vi "HFRR ADV v01.vi"() -> ()   [LabVIEW 2025] (continued)
  # "mm"
  # "°C"
  # "%RH"
  # "min"
  # "mins remaining"
  # "°C"
  # "Coefficient of Friction"
  # "Frictional Force ( N )"
  # "Electrical Contact Resistance ( % )"
  # "Temperature ( °C )"
  # "Heater"
  # "( mm )"
  # "Hz"
  # "%Rh"
  # "Stroke ( mm )"
  # "Controller"
  # "%"
  # "N"
  # "deg C"
  # "N"
  # "Automated Scar Detection in Progress"
  # "Zoom Factor"
  # "%"
  # "Tools"
  # "Wear Scar Measurements"
  # "Wear Scar"
  # "Wear Scar"
  # "Wear Scar"
  # "µm"
  # "µm"
  # "µm"
  # "Calibration Centre\nSelect a calibration procedure to begin. Each procedure guides you through all required steps."
  # "LAST CALIBRATION SESSION"
  # "Stroke"
  # "Friction"
  # "Temperature"
  # "Apply known deadweight loads to validate \nthe friction force measurement chain \nand compute the calibration factor for the f\norce transducer."
  # "Step-by-step guided displacement calibration \nacross 6 positions from 0.1 mm to 1.2 mm. Tear \nfirst, then measure each position one by one."
  # "Two-set calibration: one point at 0 °C \nice-point) and one at 60 °C (high-point) \nusing a  reference Calibrator."
  # "Step 1 — Ball Holder"
  # "Remove the ball holder by loosening and removing the center screw for stroke calibration."
  # "Step 2 — Disc Holder"
  # "Remove the disc holder by loosening and removing the screws. Clean any fluid present in the disc holder."
  # "Step 3 — Calibration Head"
  # "Place the calibration holder in position and securely tighten the center screw."
  # "Step 4 — Calibration Holder"
  # "Place the calibration holder in position and tighten the two securing screws"
  # "Step 5 — Calibration Carriage"
  # "Position the calibration carriage in the center cavity of the calibration holder and securely tighten the upper and side screws"
  # "Step 7 — Tare ( ZERO REFERENCE )"
  # "Move the carriage to the mechanical zero stop — no displacement applied. Before measuring, the sensor must be Preset. Once in position, tap Tare & Begin to zero the reference."
  # "Step 8 — POSITION MEASUREMENT"
  # "Measurement Checklist"
  # "Position the carriage at exactly this \nvalue using your reference gauge, then tap Confirm &\n Next."
  # "Positions recorded!\n\nTap Confirm & Next  to review the calibration summary."
  # "Step 9 — CALIBRATION RESULT"
  # "Stroke Calibration Complete"
  # "Calibration completed successfully. The measured stroke length is within the acceptable tolerance range of the factory calibration value."
  # "Calibration failed. The measured stroke length differs from the factory calibration value by more than 20%. Please perform the calibration again."
  # "Step 1 — Ball Holder"
  # "Remove the ball holder by loosening and removing the center screw for Friction calibration."
  # "Step 2 — Disc Holder"
  # "Remove the disc holder by loosening and removing the opposing screws. Clean any fluid present in the disc holder."
  # "Step 3 — Calibration Head"
  # "Place the calibration holder in position and securely tighten the center screw."
  # "Step 4 — Calibration Holder"
  # "Place the calibration holder in position and tighten the two securing screws"
  # "Step 5 — Tare (Spring at Free Length)"
  # "Ensure the spring is at its contact (compressed) length — the micrometer head is in contact. Click Tare Sensor to zero the friction force baseline."
  # "Step 6 — Measure Friction Force"
  # "Run the Actual Test to measure Friction Force."
  # "Calibration in Progress"
  # "Step 7 — CALIBRATION RESULT"
  # "Calibration completed successfully. The measured friction force is within the acceptable tolerance range of the factory calibration value."
  # "Calibration failed. The measured friction force differs from the factory calibration value . Please perform the calibration again."
  # "Spring Constant: k = 1.000 N/mm\nSpring force |F| = k Ч d"
  # "Calibrates the sample/bath temperature sensor. \nUsed for test specimen and lubricant temperature measurement."
  # "Calibrates the ambient air temperature sensor. \nUsed for environmental chamber monitoring."
  # "Set B\n60 °C\nHigh-point calibration"
  # "Set A\n0 °C\nIce-point calibration"
  # "Set B\n60 °C\nHigh-point calibration"
  # "Set A\n0 °C\nIce-point calibration"
  # "Select Temperature Sensor"
  # "Choose which temperature sensor you are calibrating. Both use the same two-\npoint procedure: 0 °C (ice-point) and 60 °C (high-point)."
  # "Step 1 — Reference Instrument Setup"
  # "Connect a calibrated reference to the DUT port. This calibration performs two sets: one at 0 °C and one at 60 °C."
  # "Set A\n0 °C\nIce-point calibration"
  # "Set B\n60 °C\nHigh-point calibration"
  # "Allow the temperature bath to stabilise for at least 2 minutes at each set-point before recording the reading."
  # "Step 2 — Set A:  0 °C Calibration"
  # "Connect the  0 °C reference connector. Wait for the temperature to stabilise. Once stable, and click Record Point."
  # "Step 3 — Set B:  60 °C Calibration"
  # "Connect the  60 °C reference connector. Wait for the temperature to stabilise. Once stable, and click Record Point."
  # "Sample Temperature Calibration Complete"
  # "Sample Temperature Calibration PASSED\nMax deviation 0.200 °C — within ±0.5 °C tolerance. Two-point correction applied (0 °C & 60 °C)."
  # "Sample  Temperature Calibration Failed\nmeasured Sample Temperature differs from the factory calibration value"
  # "Step 1 — Reference Instrument Setup"
  # "Connect a calibrated reference to the DUT port. This calibration performs two sets: one at 0 °C and one at 60 °C."
  # "Set A\n0 °C\nIce-point calibration"
  # "Set B\n60 °C\nHigh-point calibration"
  # "Allow the temperature bath to stabilise for at least 2 minutes at each set-point before recording the reading."
  # "Step 2 — Set A:  0 °C Calibration"
  # "Connect the  0 °C reference connector. Wait for the temperature to stabilise. Once stable, and click Record Point."
  # "Step 3 — Set B:  60 °C Calibration"
  # "Connect the  60 °C reference connector. Wait for the temperature to stabilise. Once stable, and click Record Point."
  # "Air Temperature Calibration Complete"
  # "Air Temperature Calibration PASSED\nMax deviation 0.200 °C — within ±0.5 °C tolerance. Two-point correction applied (0 °C & 60 °C)."
  # "Air  Temperature Calibration Failed\nmeasured Sample Temperature differs from the factory calibration value"
  # "PID SAVE PARAMETERS"
  # "STROKE CALIBRATION"
  # "FF CALIBRATION"
  # "ABOUT SCREEN SAVE PARAMETERS"
  # "© 2023"
  # "System Control Commands\nS;1 - Starts the full automation cycle (Runs Priming-humidify till 70RH sequence first, then switches to Maintenance).\nS;0 - Stops the system immediately and enters Standby mode (Safe State: All actuators OFF).\nM;1 - Skips the priming sequence and jumps directly to Maintenance mode (PID control).\nR;1 - Resets the logic state machine and clears all errors, returning to Standby.\nService Mode (Manual Control)\nX;1 - Enters Manual Service Mode. This disables all automatic logic, sensor safety checks, and timers.\nX;0 - Exits Manual Service Mode and returns to Standby (Safe State).\nActuator Commands (Only work after sending X;1)\nP;[0-255] - Sets the Pump PWM. Note that this is Active Low (0 = Max Flow, 255 = Pump OFF).\nF;I;[0-255] - Sets the Intake Fan speed (0 = OFF, 255 = Max Speed).\nF;O;[0-255] - Sets the Exhaust Fan speed (0 = OFF, 255 = Max Speed).\nD;1 - Turns the Dehumidifier Relay ON.\nD;0 - Turns the Dehumidifier Relay OFF."
  # "%RH"
types:
  T1 = enum32{"Home", "Dashboard", "Imaging", "Report", "Analysis", "About", "Test Setup", "Advance", "Calibration"}
  T2 = typedef "imagedata.ctl" = cluster{"image type":i32, "image depth":i32, "image":u8[], "mask":u8[], "colors":u32[], "Rectangle":cluster{"left":i16, "top":i16, "right":i16, "bottom":i16}}
  T3 = enum32{"HOME", "Test Setup", "Acquire", "Compare Files", "Print Report", "About", "Advance", "Mooha"}
  T4 = enum32{"HOME", "Test Setup", "Acquire", "Adv Scar", "Adv Scar Report", "Compare Files", "Calibration", "About", "Advance", "Mooha"}
  T5 = enum16{"ASTM D6079", "ISO 12156", "CEC F-096-A-06", "Custom"}
  T6 = enum32{"Dashboard 1", "Dashboard 2", "Dashboard 3"}
  T7 = enum32{"COF", "Friction", "ECR", "Temperature", "Stroke"}
  T8 = enum32{"Coefficient Of Friction", "Air Temperature", "Humidity", "Stroke", "Sample Temperature", "Electrical Contact Resistance", "Frequency", "Air Temp vs Rh"}
  T9 = enum32{"Main", "Stroke", "Friction", "Temperature"}
  T10 = enum32{"Stroke Calibration", "Friction Force Calibration", "Temperature Calibration", "Default"}
  T11 = enum32{"Step 1", "Step 2", "Step 3", "Step 4", "Step 5", "Step 6", "Step 7", "Step 8", "Step 9"}
  T12 = enum32{"Test Progress", "Stroke Points Completed"}
  T13 = enum32{"Page 1", "Page 2", "Page 3", "Page 4", "Page 5", "Page 6"}
  T14 = enum32{"Main", "Step 1", "Step 2", "Step 3", "Step 4", "Air Step 1", "Air Step 2", "Air Step 3", "Air Step 4"}
  T15 = enum32{"Air Temperature", "Sample Temperature", "Default"}
  T16 = enum32{"COMMUNICATION", "CALIBRATION", "Temp Variables", "Camera", "WO 2472 (1)", "WO 2472 (2)", "WO 2472 (3)"}
  T17 = typedef "Auto Start enum.ctl" = enum16{"Init", "Humidity & Temperature On", "Reach point", "Maintain Stage", "Start Stage", "close", "Exit"}
  T18 = typedef "DEMO Main Enum.ctl" = enum16{"INIT", "DEMO START", "MAIN SCREEN  ENTRY", "TEST PARAMETERS", "DASHBOARD", "IMAGING", "REPORT", "DEMO STOP"}
  T19 = cluster{"Read Heave and Surge":string, "Bytes at Heave Port":dbl, "Heave and Surge COM Port:":refnum<visa-resource-name>, "Com Port 2":refnum<visa-resource-name>, "Residual Due":string, "Heave COM Status 2":bool, "Heave COM Status":bool, "Port 2":bool, "Sway PPR":dbl, "Surge PPR":dbl, "Heave PPR":dbl, "Sway Pitch":dbl, "Surge Pitch":dbl, "Heave Pitch":dbl, "Sway Pulses/mm":dbl, "Surge Pulses/mm":dbl, "Heave Pulses/mm":dbl, "inner loop":dbl, "Read Heave and Surge 2":string, "String 36":string, "Write S":bool, "WriteCC1":string[], "Heave COM Loop":i32, "LastCom":string, "EXIT":bool, "Error Heave":errorcluster}
  T20 = enum8{"Enabled", "Disabled", "Disabled and Grayed Out"}
  T21 = cluster{"Read Uno":string, "Bytes at Heave Port":dbl, "UNO COM Port:":refnum<visa-resource-name>, "UNO COM Port: 2":refnum<visa-resource-name>, "Residual Due":string, "UNO COM Status 2":bool, "UNO COM Status":bool, "Port 2":bool, "Sway PPR":dbl, "Surge PPR":dbl, "Heave PPR":dbl, "Sway Pitch":dbl, "Surge Pitch":dbl, "Heave Pitch":dbl, "Sway Pulses/mm":dbl, "Surge Pulses/mm":dbl, "Heave Pulses/mm":dbl, "inner loop":dbl, "Read Heave and Surge 2":string, "String 36":string, "Write S":bool, "WriteCC1":string[], "Heave COM Loop":i32, "LastCom":string, "EXIT":bool, "Error Heave":errorcluster}
  T22 = enum32{"HOME", "Test Setup", "Acquire", "Adv Scar", "Adv Scar Report", "Compare Files", "About", "Advance", "Mooha"}
  T23 = typedef "POST ANALYSIS ENUM.ctl" = enum16{"OPEN EXE", "INIT", "OPEN FILE", "FIT", "DRAW REC", "DRAW LINE", "PAN", "ZOOM IN", "ZOOM OUT", "SET ZOOM", "CLEAR ROI", "GET MEASUREMENTS", "RESIZE MODE", "STREAM START", "STREAM STOP", "SHOW UI", "MINIMIZE UI", "HIDE UI", "CKISE APP", "CLOSE CONNECTION", "SAVE IMAGE", "SET ROI COLOR", "READ", "TCP CHECK", "CLOSE"}
  T24 = typedef "CAMERA LIVE FEED ENUM.ctl" = enum16{"OPEN EXE", "INIT", "READ", "CAMERA CONNECT", "CAMERA START", "CAMERA STOP", "CAMERA GRAY", "CAMERA RGB", "CAMERA MINIMIZE", "CAMERA CLOSE", "CAMERA MODE LIST", "CAMERA MODE SET", "CAMERA RESTORE", "CAMERA SAVE", "CLOSE"}
  T25 = enum16{"Always On", "Always Off", "Off While Running"}
  T26 = enum32{"Home", "Dashboard", "Imaging", "Report", "Analysis", "About", "Test Setup", "Advance"}
  T27 = cluster{"File Name":string, "Test Method":string, "Operator":string, "Fuel Description":string, "Date and time":string}
  T28 = enum32{"Home", "Dashboard", "Imaging", "Report", "Analysis", "About", "Test Setup"}
  T29 = enum32{"HOME", "Test Setup", "Acquire", "Compare Files", "About", "Advance", "Mooha"}
  T30 = typedef "NI_ReportGenerationCore.lvlib/HTML Report Image Alignment.ctl" = enum16{"(default)", "LEFT", "RIGHT", "TOP", "TEXTTOP", "MIDDLE", "ABSMIDDLE", "BASELINE", "BOTTOM", "ABSBOTTOM"}
  T31 = cluster{"y":dbl, "LVDT STROKE DISPLAY":dbl, "y":dbl}
  T32 = enum16{"INIT", "READ", "MANUAL WRITE", "WRITE", "CLOSE", "ERROR INIT"}
diagram:
  w2 = FALSE
  w9 = 0.0 ("ch0_filt")
  w11 = -9999999.0 ("max_ch0")
  w12 = 9999999.0 ("min_ch0")
  w23 = FALSE ("Visible")
  w24 = T20."Enabled" ("Disabled")
  w27 = FALSE ("Visible")
  w26 = FALSE ("Humidity Off Command")
  w42 = "" ("USER ID")
  (unwired) T22."HOME" ("Main Tab")
  # "Temperature Continue Air Step 2"
  # "[CH1]    - FF\n[CH2]   - TEMPERATURE\n[CH3]    - Humidity\n[CH4]    - AIR TEMP\n[CH5]\\- Visa Uno\n[CH6] \\- Visa Due\n[CH7]  \\- file path\n[CH8]   - Displacement Gain\n[CHA]   - Stroke Gain\n[CHB]   - Stroke PID Gain\n[CHC]   -Language Selection\n[CHD]   -Power +\n[CHE]   -Power_\n[CHF]   -Heater\n[CHG]   -Humidity Wet\n[CHH]   -Humidity Dry\n[CHI]   -Integral Time \n[CHIJ   -Air intercept\n[CHI]   -Temp Intercept"
  n1 = local write "Cal Password"("" ("Cal Password")) -> ()
  n2 = property on="Auto Start Test" class="Bool (strict)"("Visible"=TRUE) -> ()  [unwired: 2 in, 2 out]
  n3 = property on="Friction Force Calibration Result Tab" class="TabCtl (strict)"("Visible"=FALSE) -> ()  [unwired: 2 in, 2 out]
  n4 = property on="FRICVALZ 2" class="Bool (strict)"("DisabledEnum"=w24) -> ()  [unwired: 2 in, 2 out]
  n5 = property on="FRICVALZ 4" class="Bool (strict)"("DisabledEnum"=w24) -> ()  [unwired: 2 in, 2 out]
  n6 = property on="FRICVALZ 3" class="Bool (strict)"("DisabledEnum"=w24) -> ()  [unwired: 2 in, 2 out]
  n7 = property on="About" class="Clust (strict)"("Visible"=FALSE) -> ()  [unwired: 2 in, 2 out]
  n8 = property on="Wrong Password" class="Str"("Visible"=w23) -> ()  [unwired: 2 in, 2 out]
  n9 = property on="Calibration 2" class="TabCtl (strict)"("Visible"=w23) -> ()  [unwired: 2 in, 2 out]
  n10 = local write "Temperature Selection"(T15."Default" ("Temperature Selection")) -> ()
  n11 = local write "Calibration Selection"(T10."Default" ("Calibration Selection")) -> ()
  n12 = local write "SCAR MEASURMENT"(enum32{"Auto Scar", "Manual Scar"}."Manual Scar" ("SCAR MEASURMENT")) -> ()
  n13 = property on="Service Left" class="Bool (strict)"("Visible"=w2) -> ()  [unwired: 2 in, 2 out]
  n14 = property on="Service Right" class="Bool (strict)"("Visible"=w2) -> ()  [unwired: 2 in, 2 out]
  n15 = property on="Service Bottom" class="Bool (strict)"("Visible"=w2) -> ()  [unwired: 2 in, 2 out]
  n16 = flat-sequence {
    tunnel: [w78] -> w8
    tunnel: [w123] -> w34
    tunnel: w8 -> [w118]
    tunnel: [w124] -> w36
    tunnel: w34 -> [w124]
    tunnel: w36 -> [w184]
    tunnel: [w184] -> w35
    tunnel: w35 -> [w215]
    tunnel: [w215] -> w45
    tunnel: w45 -> [w222]
    tunnel: [w228] -> w33
    tunnel: [w216] -> w32
    tunnel: [w270] -> w7
    tunnel: [w269] -> _
    tunnel: w33 -> [w269]
    tunnel: w32 -> [w270]
    frame #0 {
      n17 = call "CLOSE CONNECTION.vi"("error in (no error)"="error in (no error) 2") -> ("error out"=w83:errorcluster)  [unwired: 10 in]
      n18 = call <vilib>:"Clear Errors.vi"("error in (no error)"=w83) -> ("error out"=w82:errorcluster)  [unwired: 5 in, 1 out]
      n19 = disable-structure shown="Enabled" {
        disable-tunnel: w82 -> [w110 _]
        disable-tunnel: [w109 _] -> w81
        frame Enabled {
          n20 = call <userlib>:"Fit VI window to Largest Dec.vi"("error in (no error)"=w110, "border spacing (2 px)"=1) -> ("error out"=w113:errorcluster, "dup VI Ref"=w117:refnum<vi>)  [unwired: 4 in]
          n21 = invoke on="Invoke Node" class="VI" method="FP.Run-Time Position.Maximized"(reference=w117, error in=w113) -> (error out=w114:errorcluster)  [unwired: 2 in, 3 out]
          n22 = call <vilib>:"Clear Errors.vi"("error in (no error)"=w114) -> ("error out"=w116:errorcluster)  [unwired: 5 in, 1 out]
          n23 = control-ref of="This VI"() -> (w108:refnum<vi>)
          n24 = invoke on="Invoke Node" class="VI" method="Default Vals.Reinit All"(reference=w108, error in=w116) -> (reference out=w112:refnum<vi>, error out=w111:errorcluster)  [unwired: 1 in, 1 out]
          n25 = Close Reference(reference=w112, error in (no error)=w111) -> (error out=w109:errorcluster)
        }
        frame Disabled {
        }
      }
      n26 = call "Stall Data Flow.vim"("value in"=w81, "milliseconds to wait"=u32 2000) -> ("value out"=w80:errorcluster)  [unwired: 1 out]
      n27 = call "Read Config.vi"("error in (no error)"=w80) -> ("error out"=w78:errorcluster, "STROKE PARAMETERS"=w89:dbl[], "ADC PARAMETERS"=w90:dbl[], "PID  PARAMETERS"=w91:dbl[], "CALIBRATION PARAMETERS"=w76:string[], "Stroke Calibration"=w88:string)  [unwired: 5 in]
      n28 = Index Array(array=w76) -> (element #1=w75:string, element #2=w74:string, element #3=w73:string, element #4=w72:string, element #5=w71:string, element #6=w69:string, element #7=w68:string, element #8=w67:string, element #9=w66:string, element #10=w65:string, element #11=w64:string, element #12=w63:string)  [unwired: 12 in]
      n29 = Index Array(array=w89) -> (element #1=w106:dbl, element #2=w107:dbl)  [unwired: 2 in]
      n30 = Index Array(array=w90) -> (element #1=w102:dbl, element #2=w103:dbl, element #3=w104:dbl, element #4=w105:dbl, element #5=w70:dbl)  [unwired: 5 in]
      n31 = Index Array(array=w91) -> (element #1=w93:dbl, element #2=w94:dbl, element #3=w95:dbl, element #4=w96:dbl, element #5=w97:dbl, element #6=w98:dbl, element #7=w99:dbl, element #8=w100:dbl, element #9=w101:dbl)  [unwired: 9 in]
      n32 = local write "STROKE FILTER"(w106) -> ()
      n33 = local write "Add up Stroke"(w107) -> ()
      n34 = local write "milliseconds to wait"(w93) -> ()
      n35 = local write "dt"(w94) -> ()
      n36 = local write "kp"(w95) -> ()
      n37 = local write "ki"(w96) -> ()
      n38 = local write "kd"(w97) -> ()
      n39 = local write "max_step_change"(w98) -> ()
      n40 = local write "max_amplitude"(w99) -> ()
      n41 = local write "min_amplitude"(w100) -> ()
      n42 = local write "startup_cmd"(w101) -> ()
      n43 = local write "VREF"(w102) -> ()
      n44 = local write "ADC_Resolution"(w103) -> ()
      n45 = local write "PIEZO_CAL_FACTOR"(w104) -> ()
      n46 = local write "NORMAL_FORCE"(w105) -> ()
      n47 = local write "Machine Serial Number"(w71) -> ()
      n48 = local write "STROKE CALIBRATION"(w75) -> ()
      n49 = local write "FRICTION CALIBRATION"(w74) -> ()
      n50 = local write "TEMPERATURE CALIBRATION"(w73) -> ()
      n51 = Fract/Exp String To Number(string=w72) -> (number=w77:dbl)  [unwired: 3 in, 1 out]
      n52 = local write "FF CAL EXCPTED VALUE"(w70) -> ()
      n53 = local write "version"(w69) -> ()
      n54 = local write "Version"(w68) -> ()
      n55 = local write "Workorder"(w67) -> ()
      n56 = local write "Runtime"(w66) -> ()
      n57 = local write "Firmware Version"(w65) -> ()
      n58 = local write "Operating System"(w64) -> ()
      n59 = local write "Instrument Serial"(w63) -> ()
      n60 = Spreadsheet String To Array(delimiter (Tab)=";", format string="", spreadsheet string=w88, array type (2D Dbl)=dbl[] []) -> (array=w92:dbl[])
      n61 = local write "Temperature diff"(w77) -> ()
      n62 = local write "calibration values"(w92) -> ()
    }
    frame #1 {
      n63 = property on="Auto Scar Check" class="Clust (strict)"("Visible"=TRUE) -> ()  [unwired: 2 in, 2 out]
      n64 = property on="Sign In" class="Bool (strict)"("DisabledEnum"=T20."Disabled" ("Disabled")) -> ()  [unwired: 2 in, 2 out]
      n65 = local write "sign in temp"(FALSE ("sign in temp")) -> ()
      n66 = call "dialog box.vi"("Status"="Before starting the test, verify that the microscope cable is connected.", "error in"=w118) -> ("error out"=w123:errorcluster)  [unwired: 8 in]
    }
    frame #2 {
      (unwired) TRUE ("Re-Initialise")
      # "kkkkk"
      # "C:\\Windows\\wndcm_pw_stdED hfrr.txt"
      # "C:\\LAB-IQ NXT"
      # "C:\\LAB-IQ NXT\\wndcm_pw_stdED hfrr.txt"
      # "password file"
      n67 = Current VI's Path() -> (path=w140:path)
      n68 = Strip Path(path=w140) -> (stripped path=w133:path)  [unwired: 1 out]
      n69 = local write "main tab sub"(enum32{"Page 1", "Page 2"}."Page 1" ("main tab sub")) -> ()
      n70 = local write "Main Tab Display"(T6."Dashboard 1" ("Main Tab Display")) -> ()
      n71 = local write "Main Tab"(T4."HOME" ("Main Tab")) -> ()
      n72 = Path To String(path=w133) -> (string=w135:string)
      n73 = Search/Split String(string=w135, search string/char (-)=".exe") -> (match + rest of string=w137:string)  [unwired: 1 in, 2 out]
      n74 = Match True/False String(2:".vi" ("false string"), 3:".exe" ("true string"), 4:w137) -> (0:w134:bool)  [unwired: 1 out]
      n75 = List Folder(path=path "C:/LAB-IQ" ("directory path"), pattern="*.txt") -> (filenames=w146:string[])  [unwired: 2 in, 3 out]
      n76 = case shown="True" w134 {
        tunnel: w133 -> [w155 w157]
        tunnel: [w155 w156] -> w131
        frame False {
        }
        frame True {
          n77 = Strip Path(path=w157) -> (stripped path=w156:path)  [unwired: 1 out]
        }
      }
      n78 = Search 1D Array(1D array=w146, element="wndcm_pw_stdED hfrr.txt") -> (index of element=w149:i32)  [unwired: 1 in]
      n79 = Equal?(x=w149, y=-1) -> (x = y?=w144:bool)
      n80 = Path To String(path=w131) -> (string=→"Gain path":string)
      n81 = case shown="True" w144 {
        frame False {
        }
        frame True {
          n82 = String To Byte Array(string="123\n") -> (unsigned byte array=w162:u8[])
          n83 = Array Size(array=w162) -> (size(s)=w161:i32)
          n84 = for {
            N: w161 -> [_]
            tunnel: w162 -> [w175]
            tunnel: [w172] -> w164 mode=indexing
            tunnel: w161 -> [w167]
            i -> [w165]
            n85 = Decrement(x=w167) -> (x-1=w168:i32)
            n86 = Index Array(array=w175, index=w165) -> (element=w174:u8)
            n87 = Equal?(x=w165, y=w168) -> (x = y?=w169:bool)
            n88 = Number To Decimal String(number=w174) -> (decimal integer string=w173:string)  [unwired: 1 in]
            n89 = Select(t="", s=w169, f="\r") -> (s? t:f=w166:string)
            n90 = Concatenate Strings(w173, w166) -> (w172:string)
          }
          n91 = local read "file path"() -> (w158:path)
          n92 = Concatenate Strings(w164) -> (w160:string)
          n93 = call <vilib>:"Write Characters To File.vi"("append to file? (new file:F)"=FALSE, "character string"=w160, "file path (dialog if empty)"=w158) -> ()  [unwired: 2 in, 1 out]
        }
      }
      n94 = local write "conststatus"(0.0 ("rpm value : 2")) -> ()
      n95 = local write "EVENT LOG"("") -> ()
      n96 = local write "COUNT"(0 ("COUNT")) -> ()
      n97 = local write "clk"(0.0 ("clk")) -> ()
      n98 = local write "Flag"(0.0 ("Flag")) -> ()
      n99 = local write "Lan flag"(0.0 ("Lan flag")) -> ()
      n100 = local write "Com flag"(u32 0 ("Com flag")) -> ()
      n101 = local write "refresh flag"(FALSE ("refresh flag")) -> ()
      "file path" <- path "C:/LAB-IQ/wndcm_pw_stdED hfrr.txt" ("file path")
      "FF buffer" <- dbl[] [] ("FF buffer")
    }
    frame #3 {
      # "C:\\WinDucom\\calibrate WO 2391.dcf"
      n102 = String To Path(string="C:\\LAB-IQ\\Image Calibrate v01.dcf") -> (path=w179:path)
      n103 = String To Path(string="C:\\LAB-IQ\\calibrate WO 2472.dcf") -> (path=w183:path)
      n104 = Open/Create/Replace File "Open File"(file path (use dialog)=w183) -> (refnum out=w182:refnum<file>)  [unwired: 5 in, 2 out]
      n105 = Open/Create/Replace File ("Open File")(file path (use dialog)=w179) -> (refnum out=w178:refnum<file>)  [unwired: 5 in, 2 out]
      n106 = for {
        N: 4 -> [_]
        tunnel: w178 -> [w190]
        i -> [w186]
        n107 = Read from Text File ("Read File")(file (use dialog)=w190) -> (text=w191:string)  [unwired: 3 in, 3 out]
        n108 = String Subset(string=w191, offset (0)=6, length (rest)=10 ("length (rest)")) -> (substring=w187:string)
        n109 = Fract/Exp String To Number(string=w187) -> (number=w185:dbl)  [unwired: 3 in, 1 out]
        n110 = case shown="3" w186 {
          tunnel: w185 -> [w192 w193 _ w194 _]
          frame 0 {
            n111 = local write "5x Gain"(w192) -> ()
          }
          frame 1 {
            n112 = local write "10x Gain"(w193) -> ()
          }
          frame 2 {
          }
          frame 3 {
            n113 = local write "100x gain"(w194) -> ()
          }
          frame 4, Default {
          }
        }
      }
      n114 = for {
        N: 24 -> [_]
        tunnel: w182 -> [w203]
        i -> [w197]
        (unwired) TRUE ("line mode (F)")
        n115 = Read from Text File "Read File"(file (use dialog)=w203) -> (text=w202:string)  [unwired: 3 in, 3 out]
        n116 = Match Pattern(string=w202, regular expression="]") -> (after substring=w200:string)  [unwired: 1 in, 3 out]
        n117 = String Subset(string=w202, offset (0)=5, length (rest)=10 ("length (rest)")) -> (substring=w195:string)
        n118 = Fract/Exp String To Number(string=w195) -> (number=w196:dbl)  [unwired: 3 in, 1 out]
        n119 = Match Pattern(string=w200, regular expression="-") -> (before substring=w198:string)  [unwired: 1 in, 3 out]
        n120 = case shown="18" w197 {
          tunnel: w196 -> [_ _ _ _ _ _ _ _ _ _ w210 _ _ _ _ _ _ _ _ _ _ _ _ _ _]
          tunnel: w198 -> [_ _ _ _ w206 w207 w208 _ _ _ _ _ _ _ _ _ _ _ _ _ w211 _ w212 w213 _]
          frame 0 {
          }
          frame 1 {
          }
          frame 2 {
          }
          frame 3 {
          }
          frame 4 {
            n121 = local write "Com Port 1"(w206) -> ()
          }
          frame 5 {
            n122 = local write "Com Port 2"(w207) -> ()
            n123 = local write "visa due"(w207) -> ()
          }
          frame 6 {
            n124 = String To Path(string=w208) -> (path=w209:path)
            n125 = local write "File Path"(w209) -> ()
          }
          frame 7 {
          }
          frame 8 {
          }
          frame 9 {
          }
          frame 10 {
            n126 = local write "Language Selection"(w210) -> ()
          }
          frame 11 {
          }
          frame 12 {
          }
          frame 13 {
          }
          frame 14 {
          }
          frame 15 {
          }
          frame 16 {
          }
          frame 17 {
          }
          frame 18 {
          }
          frame 21 {
          }
          frame 22 {
            n127 = local write "Com Port 3"(w211) -> ()
          }
          frame 23 {
          }
          frame 19 {
            n128 = local write "C3 :"(w212) -> ()
          }
          frame 20 {
            n129 = local write "Camera Port :"(w213) -> ()
          }
          frame 24, Default {
          }
        }
      }
    }
    frame #4 {
      n130 = Wait (ms)(milliseconds to wait=u32 1000) -> ()  [unwired: 1 out]
    }
    frame #5 {
      w231 = u32 2000 ("milliseconds to wait")
      w258 = u32 2000 ("milliseconds to wait")
      n131 = call "CAMERA LIVE FEED FGV.vi"("Enum - Menu"=CAMERA_LIVE_FEED_ENUM."OPEN EXE", "error in (no error)"=w222) -> ("error out"=w264:errorcluster)  [unwired: 8 in, 1 out]
      n132 = call "IMAGE ANALYSIS.vi"("Enum"=POST_ANALYSIS_ENUM."OPEN EXE", "error in"=w222) -> ("error out"=w219:errorcluster)  [unwired: 8 in, 1 out]
      n133 = call "Stall Data Flow.vim"("value in"=w264, "milliseconds to wait"=w258) -> ("value out"=w262:errorcluster)  [unwired: 1 out]
      n134 = call "Stall Data Flow.vim"("value in"=w219, "milliseconds to wait"=u32 8000) -> ("value out"=w218:errorcluster)  [unwired: 1 out]
      n135 = call "CAMERA LIVE FEED FGV.vi"("Enum - Menu"=CAMERA_LIVE_FEED_ENUM."INIT", "error in (no error)"=w262) -> ("error out"=w260:errorcluster)  [unwired: 8 in, 1 out]
      n136 = call "IMAGE ANALYSIS.vi"("Enum"=POST_ANALYSIS_ENUM."INIT", "error in"=w218) -> ("error out"=w216:errorcluster)  [unwired: 8 in, 1 out]
      n137 = case shown="Error .." w260 {
        selector: w260 -> [w265 _]
        tunnel: [w265 _] -> w259
        frame No Error {
        }
        frame Error {
          n138 = One Button Dialog(message="Camera initialization error.\nPlease Restart the software") -> ()  [unwired: 1 in, 1 out]
        }
      }
      n139 = property on="Camera Port :" class="CmbBox"() -> ("Strings[]"=w256:string[], "Value"=w257:string)  [unwired: 2 in, 2 out]
      n140 = Search 1D Array(1D array=w256, element=w257) -> (index of element=w255:i32)  [unwired: 1 in]
      n141 = Type Cast(type=30, x=w255) -> (*(type *) &x=w253:i32)
      n142 = call "Stall Data Flow.vim"("value in"=w259, "milliseconds to wait"=w258) -> ("value out"=w235:errorcluster)  [unwired: 1 out]
      n143 = Add(x=w253, y=48) -> (x+y=w234:i32)
      n144 = call "CAMERA LIVE FEED FGV.vi"("Enum - Menu"=CAMERA_LIVE_FEED_ENUM."CAMERA CONNECT", "error in (no error)"=w235, "CAMERA PORT"=w234) -> ("error out"=w244:errorcluster)  [unwired: 7 in, 1 out]
      n145 = call "Stall Data Flow.vim"("value in"=w244, "milliseconds to wait"=u32 5000) -> ("value out"=w245:errorcluster)  [unwired: 1 out]
      n146 = call "CAMERA LIVE FEED FGV.vi"("Enum - Menu"=CAMERA_LIVE_FEED_ENUM."CAMERA MODE LIST", "error in (no error)"=w245) -> ("error out"=w247:errorcluster)  [unwired: 8 in, 1 out]
      n147 = call "Stall Data Flow.vim"("value in"=w247, "milliseconds to wait"=w231) -> ("value out"=w246:errorcluster)  [unwired: 1 out]
      n148 = call "CAMERA LIVE FEED FGV.vi"("Enum - Menu"=CAMERA_LIVE_FEED_ENUM."READ", "error in (no error)"=w246) -> ("error out"=w233:errorcluster, "data out"=→"Camera List":string)  [unwired: 8 in]
      n149 = Type Cast(type=30, x=0) -> (*(type *) &x=w227:i32)
      n150 = call "Stall Data Flow.vim"("value in"=w233, "milliseconds to wait"=w231) -> ("value out"=w232:errorcluster)  [unwired: 1 out]
      n151 = Add(x=w227, y=48) -> (x+y=w225:i32)
      n152 = call "CAMERA LIVE FEED FGV.vi"("Enum - Menu"=CAMERA_LIVE_FEED_ENUM."CAMERA MODE SET", "error in (no error)"=w232, "CAMERA MODE"=w225) -> ("error out"=w229:errorcluster)  [unwired: 7 in, 1 out]
      n153 = call "Stall Data Flow.vim"("value in"=w229, "milliseconds to wait"=u32 2000) -> ("value out"=w249:errorcluster)  [unwired: 1 out]
      n154 = call "CAMERA LIVE FEED FGV.vi"("Enum - Menu"=CAMERA_LIVE_FEED_ENUM."CAMERA START", "error in (no error)"=w249) -> ("error out"=w250:errorcluster)  [unwired: 8 in, 1 out]
      n155 = call "Stall Data Flow.vim"("value in"=w250, "milliseconds to wait"=u32 1000) -> ("value out"=w251:errorcluster)  [unwired: 1 out]
      n156 = call "CAMERA LIVE FEED FGV.vi"("Enum - Menu"=CAMERA_LIVE_FEED_ENUM."CAMERA MINIMIZE", "error in (no error)"=w251) -> ("error out"=w228:errorcluster)  [unwired: 8 in, 1 out]
    }
    frame #6 {
      n157 = case shown="No Error" w269 {
        frame No Error {
          n158 = property on="Auto Scar Check" class="Clust (strict)"("Visible"=FALSE) -> ()  [unwired: 2 in, 2 out]
        }
        frame Error {
        }
      }
      n159 = property on="Sign In" class="Bool (strict)"("DisabledEnum"=T20."Enabled" ("Disabled")) -> ()  [unwired: 2 in, 2 out]
      n160 = local write "sign in temp"(TRUE ("sign in temp")) -> ()
    }
  }
  n161 = local write "Temperature Off Command"(w26) -> ()
  n162 = local write "Main Dashboard Buttons"(T1."Home" ("Main Dashboard Buttons")) -> ()
  n163 = property on="Tab Control 6" class="TabCtl (strict)"("Visible"=FALSE) -> ()  [unwired: 2 in, 2 out]
  n164 = local write "Humidity Off Command"(w26) -> ()
  n165 = local write "CAMERA ROI MIN TEMP"(w26) -> ()
  n166 = local write "TEST FILE NAM,E SAVED"(w26) -> ()
  n167 = local write "LIVE FEED MIN TEMP"(w26) -> ()
  n168 = local write "SCAR MEASURMENT"(enum32{"Auto Scar", "Manual Scar"}."Manual Scar" ("SCAR MEASURMENT")) -> ()
  n169 = local write "Auto stop temp"(w27) -> ()
  n170 = local write "main tab sub"(enum32{"Page 1", "Page 2"}."Page 1" ("main tab sub")) -> ()
  n171 = local write "USERNAME"(w42) -> ()
  n172 = local write "Main Tab"(T4."HOME" ("Main Tab")) -> ()
  n173 = local write "USER ID"(w42) -> ()
  n174 = property on="Auto Scar Check  2" class="Clust (strict)"("Visible"=w27) -> (error out=w30:errorcluster)  [unwired: 2 in, 1 out]
  n175 = property on="Quit" class="Bool (strict)"("Value"=FALSE ("Quit")) -> (error out=w44:errorcluster)  [unwired: 2 in, 1 out]
  n176 = while {
    stop <- w284 stop-if-true
    n177 = local read "Ambient Temperature"() -> (w282:dbl)
    n178 = Wait (ms)(milliseconds to wait=u32 200) -> ()  [unwired: 1 out]
    n179 = local read "Sample Temperature 2"() -> (w281:dbl)
    n180 = local write "Sensor value"(w282) -> ()
    n181 = local write "Sensor value"(w282) -> ()
    n182 = local write "Sensor value"(w281) -> ()
    n183 = local write "Sensor value"(w281) -> ()
    n184 = local write "Temperature — Live (Set A: 0 °C)"(w282) -> ()
    n185 = local write "Temperature — Live (Set A: 60 °C)"(w282) -> ()
    n186 = local write "Temperature — Live (Set A: 60 °C)"(w281) -> ()
    n187 = local write "Temperature — Live (Set A: 0 °C)"(w281) -> ()
    n188 = case shown="True" "Save Button" {
      selector: "Save Button" -> [_ w354]
      frame False {
      }
      frame True {
        n189 = Not(x=w354) -> (.not. x?=w353:bool)
        n190 = local read "Temperature diff"() -> (w350:dbl)
        n191 = local read "Machine Serial Number"() -> (w339:string)
        n192 = local read "milliseconds to wait"() -> (w386:u32)
        n193 = local write "Save Button"(w353) -> ()
        n194 = local read "max_step_change"() -> (w391:dbl)
        n195 = local read "FF CAL EXCPTED VALUE"() -> (w337:dbl)
        n196 = local read "Operating System"() -> (w330:string)
        n197 = local read "Firmware Version"() -> (w331:string)
        n198 = local read "max_amplitude"() -> (w392:dbl)
        n199 = local read "min_amplitude"() -> (w393:dbl)
        n200 = local read "Instrument Serial"() -> (w329:string)
        n201 = local read "PIEZO_CAL_FACTOR"() -> (w397:dbl)
        n202 = local read "startup_cmd"() -> (w394:dbl)
        n203 = local read "NORMAL_FORCE"() -> (w398:dbl)
        n204 = local read "ADC_Resolution"() -> (w396:dbl)
        n205 = local read "Workorder"() -> (w333:string)
        n206 = local read "Runtime"() -> (w332:string)
        n207 = local read "Version"() -> (w334:string)
        n208 = local read "version"() -> (w335:string)
        n209 = local read "kp"() -> (w388:dbl)
        n210 = local read "kd"() -> (w390:dbl)
        n211 = local read "calibration values"() -> (w401:dbl[])
        n212 = local read "dt"() -> (w387:dbl)
        n213 = local read "ki"() -> (w389:dbl)
        n214 = local read "STROKE FILTER"() -> (w399:i32)
        n215 = local read "Add up Stroke"() -> (w400:dbl)
        n216 = Number To Fractional String(number=w350) -> (F-format string=w349:string)  [unwired: 3 in]
        n217 = local read "VREF"() -> (w395:dbl)
        n218 = Insert Into Array(array=dbl[] [], new element #1=w386, new element #2=w387, new element #3=w388, new element #4=w389, new element #5=w390, new element #6=w391, new element #7=w392, new element #8=w393, new element #9=w394) -> (w402:dbl[])  [unwired: 1 in]
        n219 = Insert Into Array(array=dbl[] [], new element #1=w395, new element #2=w396, new element #3=w397, new element #4=w398, new element #5=w337) -> (w403:dbl[])  [unwired: 1 in]
        n220 = Array To Spreadsheet String(delimiter (Tab)=";", array=w401, 3:"" ("format string")) -> (spreadsheet string=w405:string)
        n221 = Insert Into Array(array=dbl[] [], new element #1=w399, new element #2=w400) -> (w404:dbl[])  [unwired: 1 in]
        n222 = Insert Into Array(array=string[] [], new element #1="STROKE CALIBRATION", new element #2="FRICTION CALIBRATION", new element #3="TEMPERATURE CALIBRATION", new element #4=w349, new element #5=w339, new element #6=w335, new element #7=w334, new element #8=w333, new element #9=w332, new element #10=w331, new element #11=w330, new element #12=w329) -> (w351:string[])  [unwired: 1 in]
        n223 = call "Write Config.vi"("Stroke Calibration"=w405, "CALIBRATION PARAMETERS"=w351, "STROKE PARAMETERS"=w404, "ADC PARAMETERS"=w403, "PID  PARAMETERS"=w402) -> ("error out"=w384:errorcluster)  [unwired: 6 in]
        n224 = call "Stall Data Flow.vim"("value in"=w384, "milliseconds to wait"=u32 2000) -> ("value out"=w385:errorcluster)  [unwired: 1 out]
        n225 = call "Read Config.vi"("error in (no error)"=w385) -> ("STROKE PARAMETERS"=w382:dbl[], "ADC PARAMETERS"=w381:dbl[], "PID  PARAMETERS"=w380:dbl[], "CALIBRATION PARAMETERS"=w345:string[], "Stroke Calibration"=w383:string)  [unwired: 5 in, 1 out]
        n226 = Index Array(array=w345) -> (element #1=w342:string, element #2=w341:string, element #3=w340:string, element #4=w344:string, element #5=w338:string, element #6=w328:string, element #7=w327:string, element #8=w326:string, element #9=w325:string, element #10=w324:string, element #11=w323:string, element #12=w322:string)  [unwired: 12 in]
        n227 = Index Array(array=w380) -> (element #1=w378:dbl, element #2=w377:dbl, element #3=w376:dbl, element #4=w375:dbl, element #5=w374:dbl, element #6=w373:dbl, element #7=w372:dbl, element #8=w371:dbl, element #9=w370:dbl)  [unwired: 9 in]
        n228 = Index Array(array=w381) -> (element #1=w369:dbl, element #2=w368:dbl, element #3=w367:dbl, element #4=w366:dbl, element #5=w336:dbl)  [unwired: 5 in]
        n229 = Index Array(array=w382) -> (element #1=w365:dbl, element #2=w364:dbl)  [unwired: 3 in, 1 out]
        n230 = Spreadsheet String To Array(delimiter (Tab)=";", format string="", spreadsheet string=w383, array type (2D Dbl)=dbl[] []) -> (array=w379:dbl[])
        n231 = local write "STROKE FILTER"(w365) -> ()
        n232 = local write "Add up Stroke"(w364) -> ()
        n233 = local write "VREF"(w369) -> ()
        n234 = local write "ADC_Resolution"(w368) -> ()
        n235 = local write "PIEZO_CAL_FACTOR"(w367) -> ()
        n236 = local write "NORMAL_FORCE"(w366) -> ()
        n237 = local write "FF CAL EXCPTED VALUE"(w336) -> ()
        n238 = local write "STROKE CALIBRATION"(w342) -> ()
        n239 = local write "FRICTION CALIBRATION"(w341) -> ()
        n240 = local write "TEMPERATURE CALIBRATION"(w340) -> ()
        n241 = Fract/Exp String To Number(string=w344) -> (number=w343:dbl)  [unwired: 3 in, 1 out]
        n242 = local write "Machine Serial Number"(w338) -> ()
        n243 = local write "version"(w328) -> ()
        n244 = local write "Version"(w327) -> ()
        n245 = local write "Workorder"(w326) -> ()
        n246 = local write "Runtime"(w325) -> ()
        n247 = local write "Firmware Version"(w324) -> ()
        n248 = local write "Operating System"(w323) -> ()
        n249 = local write "Instrument Serial"(w322) -> ()
        n250 = local write "calibration values"(w379) -> ()
        n251 = local write "milliseconds to wait"(w378) -> ()
        n252 = local write "dt"(w377) -> ()
        n253 = local write "kp"(w376) -> ()
        n254 = local write "ki"(w375) -> ()
        n255 = local write "kd"(w374) -> ()
        n256 = local write "max_step_change"(w373) -> ()
        n257 = local write "max_amplitude"(w372) -> ()
        n258 = local write "min_amplitude"(w371) -> ()
        n259 = local write "startup_cmd"(w370) -> ()
        n260 = local write "Temperature diff"(w343) -> ()
      }
    }
    n261 = local read "USER ID"() -> (w279:string)
    n262 = local read "run test Calibration"() -> (w277:bool)
    n263 = disable-structure shown="Enabled" {
      disable-tunnel: [w291 w302] -> w278
      frame Disabled {
        n264 = local read "Point 1 - 0.2 mm"() -> (w301:bool)
        n265 = local read "Point 2 - 0.4 mm"() -> (w300:bool)
        n266 = local read "Point 3 - 0.6 mm"() -> (w299:bool)
        n267 = local read "Point 4 - 0.8 mm"() -> (w298:bool)
        n268 = local read "Point 5 - 1.0 mm"() -> (w297:bool)
        n269 = local read "Point 6 - 1.2 mm"() -> (w296:bool)
        n270 = And(x=w301, y=w300) -> (x .and. y?=w295:bool)
        n271 = And(x=w299, y=w298) -> (x .and. y?=w294:bool)
        n272 = And(x=w297, y=w296) -> (x .and. y?=w292:bool)
        n273 = And(x=w295, y=w294) -> (x .and. y?=w293:bool)
        n274 = And(x=w293, y=w292) -> (x .and. y?=w291:bool)
      }
      frame Enabled {
        n275 = local read "Point 5 - 1.0 mm"() -> (w302:bool)
      }
    }
    n276 = local read "START TEMP"() -> (w276:bool)
    n277 = local write "OPERATOR ID"(w279) -> ()
    n278 = And(x=w276, y=w277) -> (x .and. y?=w275:bool)
    n279 = case shown="True" w275 {
      frame False {
        w303 = TRUE ("PAUSE")
